vi "vector_norm.vi"(1 "A":dbl[](array[numeric])) -> (0 "norm":dbl)   [LabVIEW 2011]
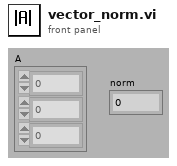
[diagram p1: front panel]
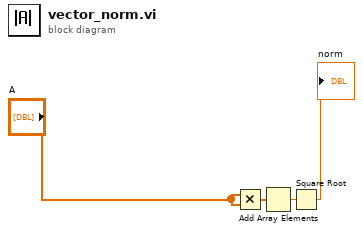
[diagram p0: block diagram]
diagram:
  n1 = Multiply(x="A", y="A") -> (x*y=w2:dbl[])
  n2 = Add Array Elements(numeric array=w2) -> (sum=w1:dbl)
  n3 = Square Root(x=w1) -> (sqrt(x)=→"norm":dbl)
